vi "TimeTool_hptime.vi"(0 "Desired Loop Time (ms)":dbl) -> (1 "elapsed time (s)":dbl, 2 "dt (ms)":dbl, 3 "error out":errorcluster)   [LabVIEW 2024]
uses:
  <vilib>/ptbypt/NI_PtbyPt.lvlib
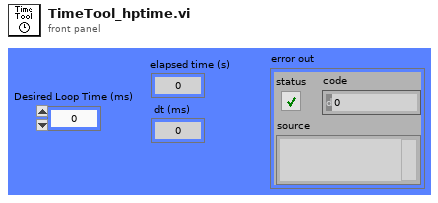
[diagram p1: front panel]
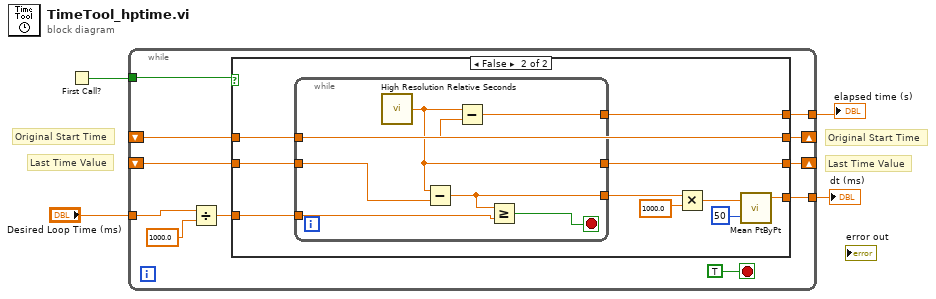
[diagram p0: block diagram]
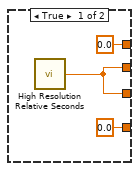
[diagram p2: hidden frame]
diagram:
  # "Last Time Value"
  # "Original Start Time"
  # "Original Start Time"
  # "Last Time Value"
  n1 = First Call?() -> (First Call?: T/F=w4:bool)
  n2 = while {
    tunnel: w4 -> [w15]
    shift-right: [w14] -> _
    shift-left: _ -> [w13]
    shift-right: [w11] -> _
    shift-left: _ -> [w10]
    tunnel: [w9] -> w3
    tunnel: [w8] -> w2
    tunnel: "Desired Loop Time (ms)" -> [w7]
    stop <- TRUE stop-if-true
    n3 = Divide(x=w7, y=1000.0) -> (x/y=w5:dbl)
    n4 = case shown="False" w15 {
      tunnel: [w18 w25] -> w14
      tunnel: w13 -> [_ w25]
      tunnel: [w18 w21] -> w11
      tunnel: w10 -> [_ w24]
      tunnel: [0.0 ("mean") w23] -> w9
      tunnel: [0.0 w20] -> w8
      tunnel: w5 -> [_ w19]
      frame True {
        n5 = call <vilib>:"High Resolution Relative Seconds.vi"() -> ("relative seconds"=w18:dbl)
      }
      frame False {
        n6 = while {
          tunnel: w25 -> [w35]
          tunnel: w24 -> [w34]
          tunnel: [w31] -> w22
          tunnel: [w33] -> w21
          tunnel: [w32] -> w20
          tunnel: w19 -> [w30]
          stop <- w29 stop-if-true
          n7 = call <vilib>:"High Resolution Relative Seconds.vi"() -> ("relative seconds"=w33:dbl)
          n8 = Subtract(x=w33, y=w34) -> (x-y=w31:dbl)
          n9 = Subtract(x=w33, y=w35) -> (x-y=w32:dbl)
          n10 = Greater Or Equal?(x=w31, y=w30) -> (x >= y?=w29:bool)
        }
        n11 = Multiply(x=w22, y=1000.0) -> (x*y=w26:dbl)
        n12 = call <vilib>:"Mean PtByPt.vi"("x"=w26, "sample length"=50 ("index")) -> ("mean"=w23:dbl)  [unwired: 2 in, 1 out]
      }
    }
  }
  "dt (ms)" <- w3
  "elapsed time (s)" <- w2
